vi "De-interleave Current Readings.vi"(10 "Input Array":dbl[](array[numeric])=[6.0, 3.9, -5.8, 0.0, -2.6, -1.0, 2.2, -4.3] format="%0.2f") -> (0 "Negative Current":dbl[](array[numeric]) format="%0.2f", 2 "Output Table":dbl[][](array[numeric]), 3 "Positive Current":dbl[](array[numeric]) format="%0.2f")   [LabVIEW 2010]
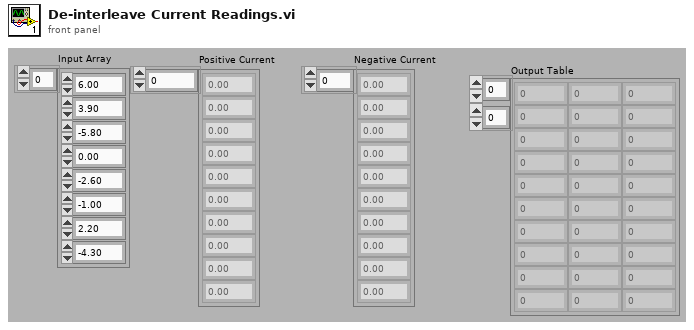
[diagram p1: front panel]
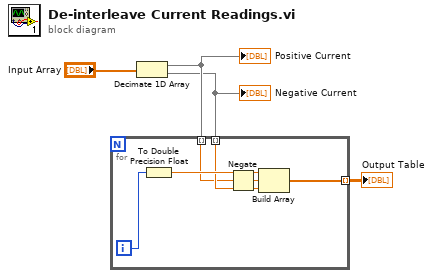
[diagram p0: block diagram]
diagram:
  n1 = Decimate 1D Array("Input Array") -> (w3:dbl[], w2:dbl[])
  "Positive Current" <- w3
  "Negative Current" <- w2
  n2 = for {
    tunnel: w3 -> [w7] mode=indexing
    tunnel: w2 -> [w8] mode=indexing
    tunnel: [w5] -> w1 mode=indexing
    i -> [w10]
    n3 = To Double Precision Float(number=w10) -> (double precision float=w9:dbl)
    n4 = Negate(x=w7) -> (-x=w6:dbl)
    n5 = Build Array(w9, w6, w8) -> (w5:dbl[])
  }
  "Output Table" <- w1
